vi "Rx Read Triggers (Pulse Output).vi"(9 "input valid (nc)":bool, 11 "niUSRP Sync":refnum<class "niUSRP Sync v1 FPGA.lvclass">, 12 "ready for output (nc)":bool, 13 "external trigger":bool) -> (10 "output valid":bool, 14 "ready for input (nc)":bool, 15 "niUSRP Sync":refnum<class "niUSRP Sync v1 FPGA.lvclass">)   [LabVIEW 2025, in "niUSRP Sync v1 FPGA.lvclass"]
doc: "this VI handles the processing of triggers and initiates the Aglinment calculation used to align Data with its corresponding Trigger. the calculation takes place before an acquisition is in progress and must be run each time the configuration changes. <b>the calculation should not be run for OTF (on the fly) changes.</b>"
uses:
  niUSRP Sync v1 FPGA.lvclass
  niUSRP Sync v1 FPGA.lvclass/niUSRP Sync v1 FPGA.ctl
  <vilib>/rvi/eio/common/nirviEmuTemplateMethod_errors.vi
  <vilib>/rvi/DataTransferAndStorage/Container/Common/niFpgaContainerExecOnDevCompGetState.vi
  <vilib>/rvi/Emulation/niFpgaEmulationIsFPGAContextNoSignature.vi
  <vilib>/rvi/DataTransferAndStorage/Container/Common/niFpgaContainerGetUniqueNameForEmu.vi
  <vilib>/rvi/Memory/Memory_Emulation/niFpgaMemoryEmulationCacheClearOnFirstRun.vi
  <vilib>/rvi/Memory/Memory_Emulation/nirvimemoryEmulationManagerCache_MakeExclusive.vi
  <vilib>/rvi/Memory/Memory_Emulation/niFpgaMemoryEmulationValidateCache.vi
  <vilib>/rvi/Memory/Memory_Emulation/nirvimemoryEmulationManagerCache_InsertValue.vi
  <vilib>/Utility/error.llb/Clear Errors.vi
  <vilib>/rvi/Memory/Memory_Emulation/nirvimemoryEmulationManagerCache_ReleaseExclusive.vi
  <vilib>/rvi/Memory/Memory_Emulation/nirvimemoryEmulationManagerCache_GetValue.vi
  <vilib>/rvi/Memory/Memory_Emulation/nirvimemoryEmulationManagerCache_SetValue.vi
  <vilib>/rvi/Emulation/niFpgaProcessEmulError.vi
  <vilib>/rvi/Emulation/niFpgaSctlEmulationGetInTimedLoop.vi
  <vilib>/eio/EIONode/EIONode.xnode
  <vilib>/rvi/DataTransferAndStorage/Container/XNode/niFpgaContainer.xnode
  <vilib>/rvi/DataTransferAndStorage/Register/Emulation/niFpgaRegisterEmulationRefIn.vi
  <instrlib>/_niInstr/Basic Elements/v1/FPGA/niInstr Basic Elements v1 FPGA.lvlib
  <instrlib>/niUsrpRio/Time/v1/FPGA/niUsrpRio Time v1 FPGA.lvlib
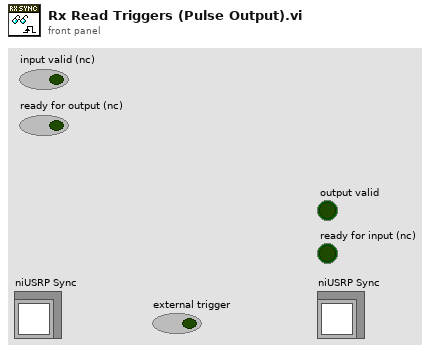
[diagram p1: front panel]
types:
  T1 = enum8{"Software", "Digital Edge", "Rx Start Trigger", "Tx Start Trigger", "Immediate", "Future Time Event"}
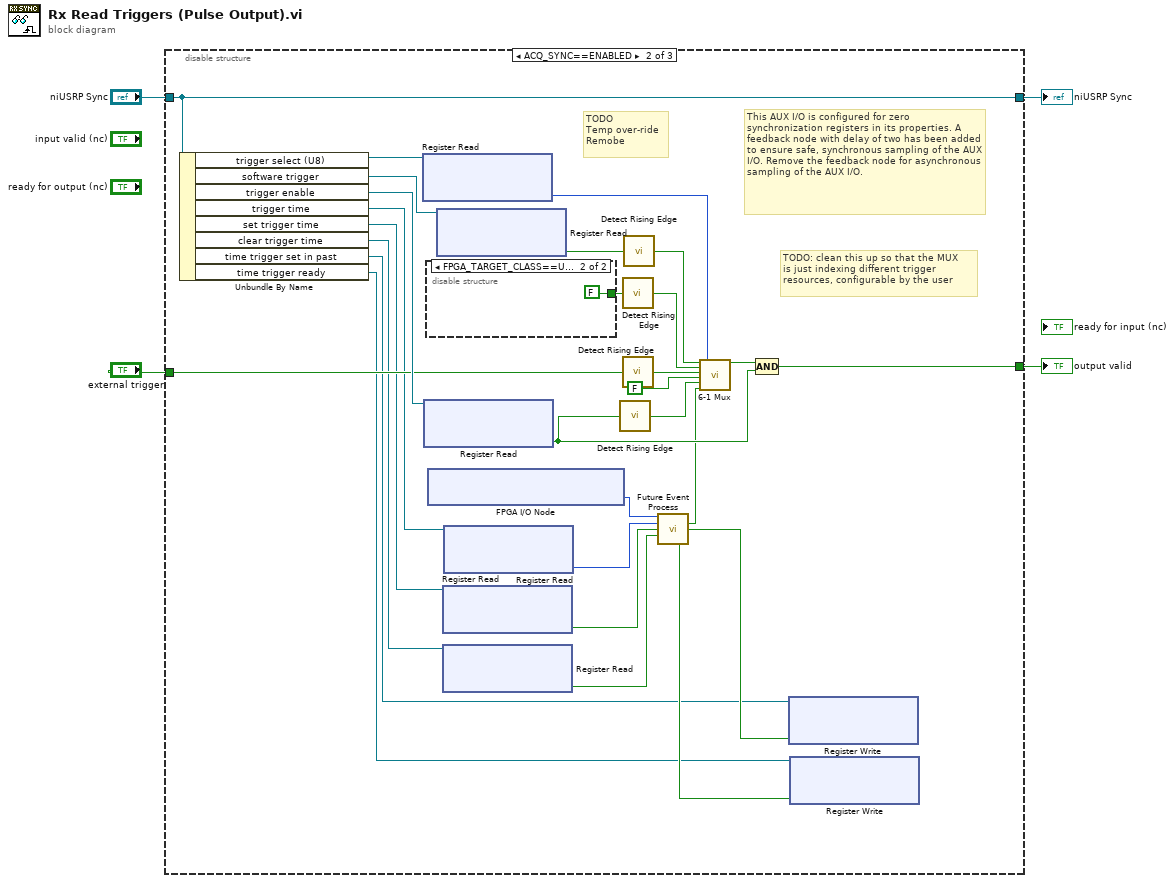
[diagram p0: block diagram]
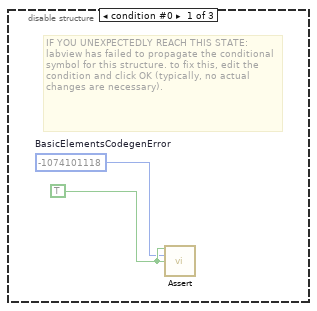
[diagram p2: hidden frame]
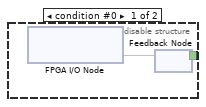
[diagram p3: hidden frame]
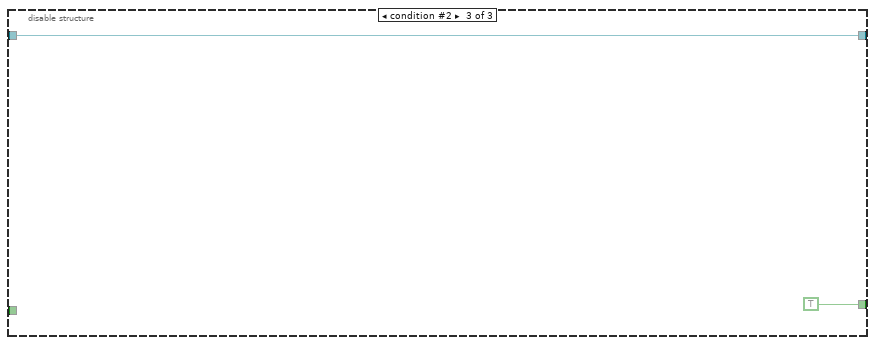
[diagram p4: hidden frame]
diagram:
  n1 = disable-structure shown="ACQ_SYNC==ENABLED" {
    disable-tunnel: "niUSRP Sync" -> [_ w24 w39]
    disable-tunnel: [_ w24 w39] -> w3
    disable-tunnel: [_ w23 TRUE] -> w2
    disable-tunnel: "external trigger" -> [_ w21 _]
    frame condition #0 {
      w6 = TRUE ("assert")
      w5 = -1074101118  # BasicElementsCodegenError
      # "IF YOU UNEXPECTEDLY REACH THIS STATE:\nlabview has failed to propagate the conditional symbol for this structure. to fix this, edit the condition and click OK (typically, no actual changes are necessary)."
      n2 = call <instrlib>:"Assert.vi"("assert"=w6, "error code"=w5, "enable show error"=w6) -> ()  [unwired: 13 in]
    }
    frame condition #1 (active) {
      # "TODO\nTemp over-ride\nRemobe"
      # "TODO: clean this up so that the MUX\nis just indexing different trigger\nresources, configurable by the user"
      # "This AUX I/O is configured for zero synchronization registers in its properties. A feedback node with delay of two has been added to ensure safe, synchronous sampling of the AUX I/O. Remove the feedback node for asynchronous sampling of the AUX I/O."
      n3 = Unbundle By Name(w24) -> ("trigger select (U8)"=w30:refnum<k21>, "software trigger"=w29:refnum<k21>, "trigger enable"=w27:refnum<k21>, "trigger time"=w12:refnum<k21>, "set trigger time"=w11:refnum<k21>, "clear trigger time"=w10:refnum<k21>, "time trigger set in past"=w9:refnum<k21>, "time trigger ready"=w8:refnum<k21>)
      n4 = xnode ("Register Read")("Register In"=w30) -> ("Data"=w19:T1)  [unwired: 1 out]
      n5 = xnode ("Register Read")("Register In"=w27) -> ("Data"=w25:bool)  [unwired: 1 out]
      n6 = disable-structure shown="FPGA_TARGET_CLASS==USRP_X410||FPGA_TARGET_CLASS==USRP_X410__EMBEDDED____UNSUPPORTED" {
        disable-tunnel: [w35 FALSE] -> w22
        frame condition #0 {
          n7 = xnode "FPGA I/O Node"() -> ("AUX I/O 0"=w36)  [unwired: 1 in, 1 out]
          n8 = feedback #1() -> (w35)  [unwired: 1 in]
          n9 = feedback-in #1(w36) -> ()
        }
        frame condition #1 (active) {
        }
      }
      n10 = xnode "FPGA I/O Node"() -> ("Daughterboard 0\\Radio Time"=w18:u64)  [unwired: 1 in, 1 out]
      n11 = xnode ("Register Read")("Register In"=w29) -> ("Data"=w28:bool)  [unwired: 1 out]
      n12 = xnode "Register Read"("Register In"=w11) -> ("Data"=w16:bool)  [unwired: 1 out]
      n13 = xnode "Register Read"("Register In"=w10) -> ("Data"=w15:bool)  [unwired: 1 out]
      n14 = xnode "Register Read"("Register In"=w12) -> ("Data"=w17:u64)  [unwired: 1 out]
      n15 = call <instrlib>:"Detect Rising Edge.vi"("signal"=w25) -> ("edge detected"=w33:bool)  [unwired: 14 in]
      n16 = call <instrlib>:"Detect Rising Edge.vi"("signal"=w22) -> ("edge detected"=w32:bool)  [unwired: 14 in]
      n17 = call <instrlib>:"Detect Rising Edge.vi"("signal"=w21) -> ("edge detected"=w20:bool)  [unwired: 14 in]
      n18 = call <instrlib>:"Detect Rising Edge.vi"("signal"=w28) -> ("edge detected"=w34:bool)  [unwired: 14 in]
      n19 = call <instrlib>:"Future Event Process.vi"("time"=w18, "future event.time"=w17, "future event.set"=w16, "future event.clear"=w15) -> ("event.occurred"=w7:bool, "future event.set in past"=w13:bool, "future event.ready"=w14:bool)  [unwired: 8 in, 1 out]
      n20 = call "6-1 Mux.vi"("input 0"=w34, "input 1"=w32, "input 2"=w20, "input 3"=FALSE ("other start trigger"), "input 4"=w33, "input 5"=w7, "select"=w19) -> ("output"=w31:bool)  [unwired: 12 in]
      n21 = Compound Arithmetic op=AND(w31, w25) -> (w23:bool)
      n22 = xnode "Register Write"("Data"=w13, "Register In"=w9) -> ()  [unwired: 1 out]
      n23 = xnode "Register Write"("Data"=w14, "Register In"=w8) -> ()  [unwired: 1 out]
    }
    frame condition #2 {
    }
  }
  "output valid" <- w2
  "niUSRP Sync" <- w3
